vi "PXI-Get Input Terminal Configuration.vi"(7 "term config in":i32(ring)=-1 items=["Default"=-1, "RSE"=10083, "NRSE"=10078, "Differential"=10106, "Pseudodifferential"=12529], 11 "error in (no error)":errorcluster, 13 "channel":string) -> (8 "term config out":i32(ring)=-1 items=["Default"=-1, "RSE"=10083, "NRSE"=10078, "Differential"=10106, "Pseudodifferential"=12529], 15 "error out":errorcluster)   [LabVIEW 2020]
uses:
  <vilib>/Utility/config.llb/Read Key (String).vi
  <vilib>/Utility/config.llb/NI_LVConfig.lvlib
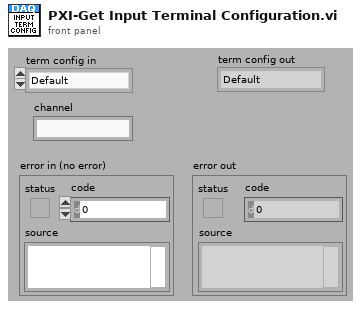
[diagram p1: front panel]
types:
  T1 = typedef "LVStringsAndValuesArrayTypeDef_I32.ctl" = cluster{"String":string, "Value":i32}[]
  T2 = typedef "NI_LVConfig.lvlib/Config Data RefNum.ctl" = refnum<k1>
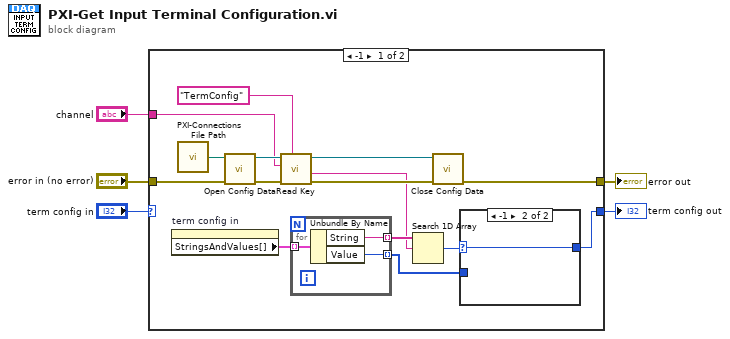
[diagram p0: block diagram]
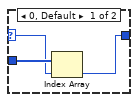
[diagram p2: hidden frame]
diagram:
  n1 = case shown="-1" "term config in" {
    selector: "term config in" -> [_ w29]
    tunnel: "error in (no error)" -> [w20 w28]
    tunnel: [w14 w28] -> w4
    tunnel: [w7 w29] -> w2
    tunnel: "channel" -> [w12 _]
    frame -1 {
      n2 = property on="term config in" class="Ring (strict)"() -> ("StringsAndValues[]"=w11:T1)  [unwired: 2 in, 2 out]
      n3 = call "PXI-Connections File Path.vi"() -> ("Path"=w13:path)  [unwired: 1 in]
      n4 = call <vilib>:"Open Config Data.vi"("error in (no error)"=w20, "configuration file path"=w13) -> ("error out"=w19:errorcluster, "refnum"=w18:T2)  [unwired: 7 in, 1 out]
      n5 = call-poly <vilib>:"Read Key.vi"("section"="TermConfig", "error in (no error)"=w19, "key"=w12, "refnum"=w18) -> ("error out"=w16:errorcluster, "value"=w9:string, "refnum out"=w15:T2)  [unwired: 4 in, 1 out]
      n6 = for {
        tunnel: w11 -> [w27] mode=indexing
        tunnel: [w26] -> w10 mode=indexing
        tunnel: [w25] -> w6 mode=indexing
        n7 = Unbundle By Name(w27) -> ("String"=w26:string, "Value"=w25:i32)
      }
      n8 = Search 1D Array(1D array=w10, element=w9) -> (index of element=w8:i32)  [unwired: 1 in]
      n9 = call <vilib>:"Close Config Data.vi"("error in (no error)"=w16, "refnum"=w15) -> ("error out"=w14:errorcluster)  [unwired: 8 in, 1 out]
      n10 = case shown="-1" w8 {
        selector: w8 -> [w22 w24]
        tunnel: [w21 w24] -> w7
        tunnel: w6 -> [w23 _]
        frame 0, Default {
          n11 = Index Array(array=w23, index=w22) -> (element=w21:i32)
        }
        frame -1 {
        }
      }
    }
    frame 1, Default {
    }
  }
  "error out" <- w4
  "term config out" <- w2
